vi "Open Instrument.vi"(8 "error in (no error)":errorcluster, 11 "Instrument.Example in":refnum<class "Instrument.LakeShore340.lvclass">) -> (0 "error out":errorcluster, 3 "Instrument.Example out":refnum<class "Instrument.LakeShore340.lvclass">)   [LabVIEW 2016, in "Instrument.LakeShore340.lvclass"]
uses:
  Instrument.LakeShore340.lvclass
  Instrument.LakeShore340.lvclass/Instrument.LakeShore340.ctl
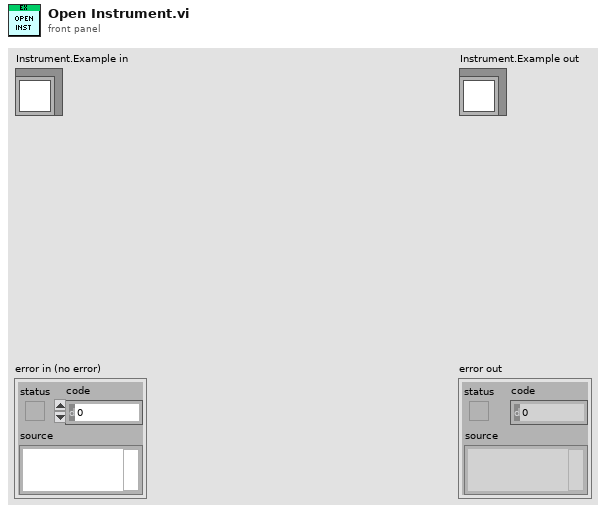
[diagram p1: front panel]
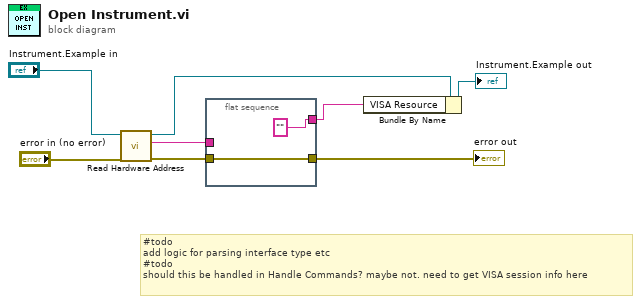
[diagram p0: block diagram]
diagram:
  # "#todo\nadd logic for parsing interface type etc\n#todo\nshould this be handled in Handle Commands? maybe not. need to get VISA session info here"
  n1 = call-dynamic "Read Hardware Address.vi"("error in (no error)"="error in (no error)", "Instrument in"="Instrument.Example in") -> ("error out"=w3:errorcluster, "Hardware Address"=w4:string, "Instrument out"=w6:refnum<class "Instrument.LakeShore340.lvclass">)  [unwired: 7 in]
  n2 = flat-sequence {
    tunnel: w4 -> [_]
    tunnel: w3 -> [w9]
    tunnel: [w9] -> w2
    tunnel: ["" ("VISA Resource")] -> w1
    frame #0 {
    }
  }
  n3 = Bundle By Name(cluster=w6, "VISA Resource"=w1) -> (→"Instrument.Example out":refnum<class "Instrument.LakeShore340.lvclass">)
  "error out" <- w2
